vi "LlegeixValorsPantalla.vi"(0 "rings":refnum<vi>[](array[refnum]), 1 "Caselles 2":refnum<vi>[](array[refnum])) -> ()   [LabVIEW 2017]
uses:
  <vilib>/registry/registry.llb/Registry RtKey.ctl
  <vilib>/registry/registry.llb/Read Registry Value Simple STR.vi
panel:
  out "Numeric":i32
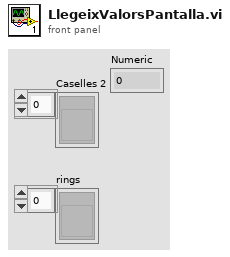
[diagram p1: front panel]
types:
  T1 = typedef "Registry RtKey.ctl" = enum32{"HKEY_CLASSES_ROOT", "HKEY_CURRENT_USER", "HKEY_LOCAL_MACHINE", "HKEY_USERS", "HKEY_PERFORMANCE_DATA", "HKEY_CURRENT_CONFIG", "HKEY_DYN_DATA"}
  T2 = typedef "Registry refnum.ctl" = refnum<k1>
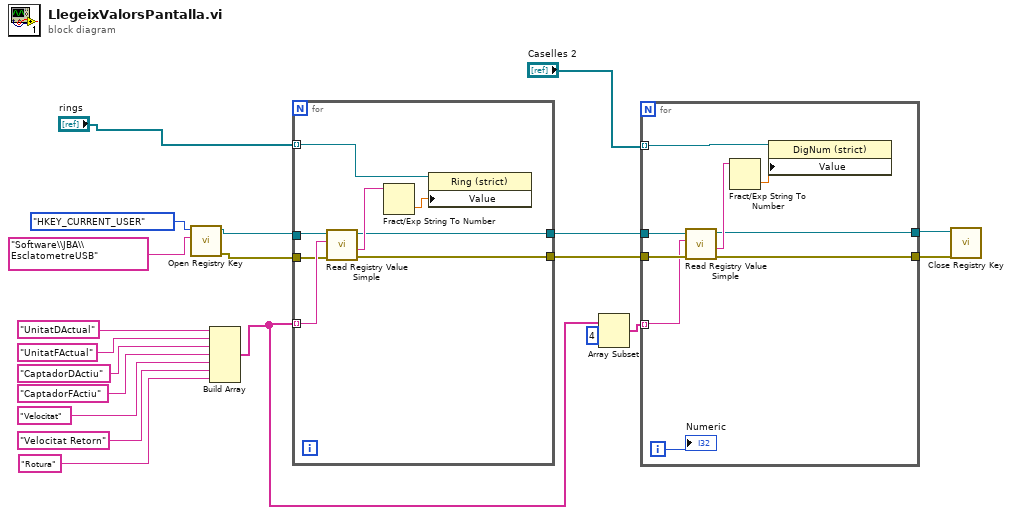
[diagram p0: block diagram]
diagram:
  n1 = call <vilib>:"Open Registry Key.vi"("subkey"="Software\\JBA\\EsclatometreUSB", "root key (HKEY_LOCAL_MACHINE)"=Registry_RtKey."HKEY_CURRENT_USER") -> ("error out"=w6:errorcluster, "refnum out"=w7:T2)  [unwired: 8 in]
  n2 = Build Array("UnitatDActual" ("value"), "UnitatFActual" ("value"), "CaptadorDActiu" ("value"), "CaptadorFActiu" ("value"), "Velocitat" ("value"), "Velocitat Retorn" ("value"), "Rotura" ("value")) -> (w11:string[])
  n3 = for {
    tunnel: "rings" -> [w28] mode=indexing
    tunnel: w11 -> [w26] mode=indexing
    tunnel: w7 -> [w27]
    tunnel: [w24] -> w10
    tunnel: [w23] -> w9
    tunnel: w6 -> [w21]
    n4 = call-poly <vilib>:"Read Registry Value Simple.vi"("error in (no error)"=w21, "value"=w26, "refnum"=w27) -> ("error out"=w23:errorcluster, "String/Binary data"=w25:string, "refnum out"=w24:T2)  [unwired: 3 in, 1 out]
    n5 = Fract/Exp String To Number(string=w25) -> (number=w22:dbl)  [unwired: 3 in, 1 out]
    n6 = property class="Ring (strict)"(reference=w28, "Value"=w22) -> ()  [unwired: 1 in, 2 out]
  }
  n7 = Array Subset(array=w11, index=4) -> (w17:string[])  [unwired: 1 in]
  n8 = for {
    tunnel: "Caselles 2" -> [w37] mode=indexing
    tunnel: w17 -> [w34] mode=indexing
    tunnel: w10 -> [w36]
    tunnel: w9 -> [w35]
    tunnel: [w31] -> w1
    tunnel: [w30] -> w2
    i -> [w29]
    n9 = call-poly <vilib>:"Read Registry Value Simple.vi"("error in (no error)"=w35, "value"=w34, "refnum"=w36) -> ("error out"=w30:errorcluster, "String/Binary data"=w32:string, "refnum out"=w31:T2)  [unwired: 3 in, 1 out]
    n10 = Fract/Exp String To Number(string=w32) -> (number=w33:dbl)  [unwired: 3 in, 1 out]
    n11 = property class="DigNum (strict)"(reference=w37, "Value"=w33) -> ()  [unwired: 1 in, 2 out]
    "Numeric" <- w29
  }
  n12 = call <vilib>:"Close Registry Key.vi"("error in (no error)"=w2, "refnum"=w1) -> ()  [unwired: 5 in, 1 out]
